vi "gpz1.vi"(8 "Y(k-2)":dbl, 9 "Y(k-1)":dbl, 10 "C(k-2)":dbl, 11 "C(k)":dbl) -> (2 "Y(k)":dbl)   [LabVIEW 2019]
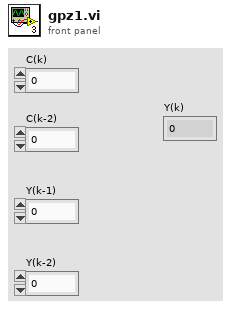
[diagram p1: front panel]
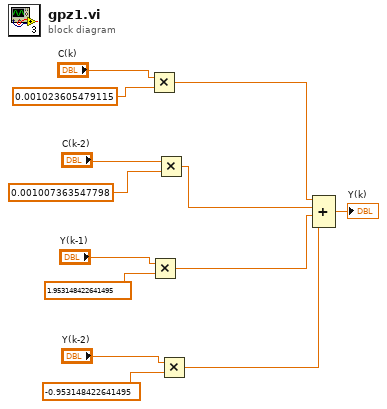
[diagram p0: block diagram]
diagram:
  n1 = Multiply(x="C(k)", y=0.001023605479115) -> (x*y=w12:dbl)
  n2 = Multiply(x="Y(k-1)", y=1.953148422641495) -> (x*y=w10:dbl)
  n3 = Multiply(x="C(k-2)", y=0.001007363547798) -> (x*y=w11:dbl)
  n4 = Multiply(x="Y(k-2)", y=-0.953148422641495) -> (x*y=w9:dbl)
  n5 = Compound Arithmetic op=ADD(w12, w11, w10, w9) -> (→"Y(k)":dbl)
